vi "rampa_lab2.vi"() -> ()   [LabVIEW 2025]
uses:
  <vilib>/Utility/file.llb/Write Delimited Spreadsheet (DBL).vi
panel:
  out "Bajo":dbl
  out "Alto":dbl
  in  "DC":dbl
  out "Waveform Chart":dynamicdata(graph)
  out "Thermometer":dbl(slide) scale=0.0..100.0
  in  "stop":bool
  # "Duty Cycle [%]"
  # "ALTO:"
  # "BAJO:"
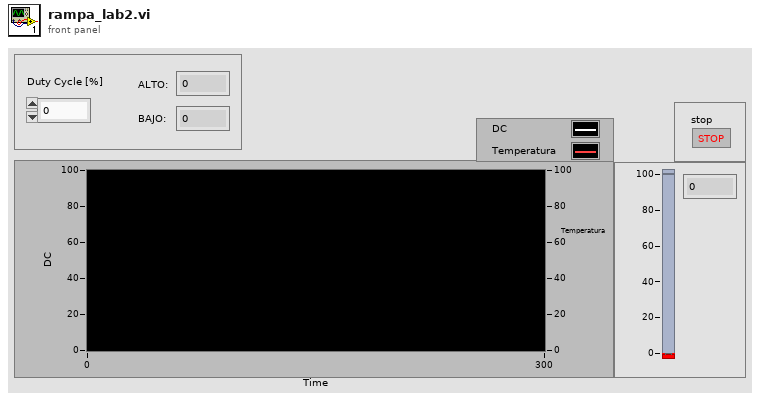
[diagram p1: front panel]
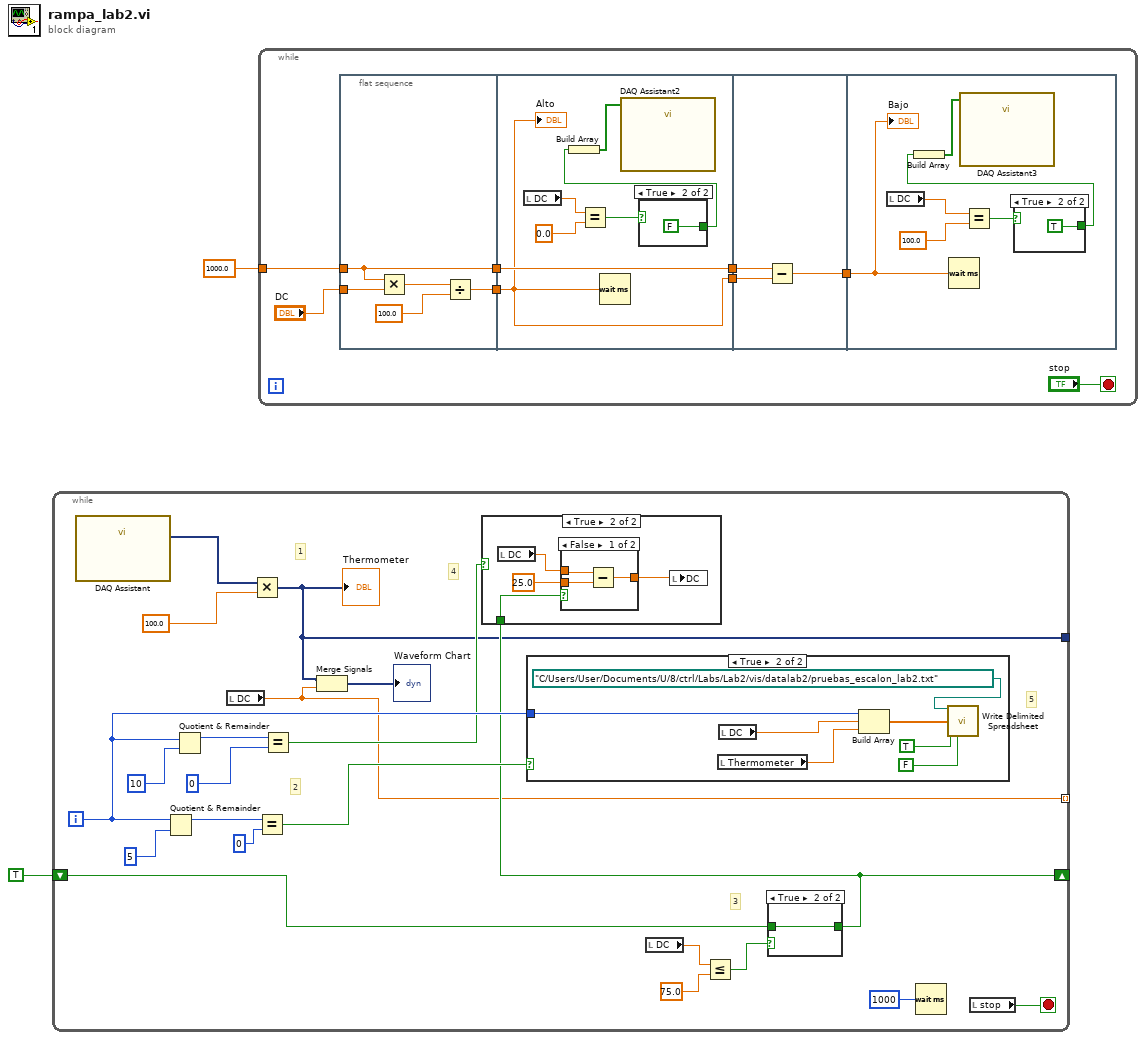
[diagram p0: block diagram]
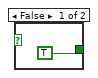
[diagram p2: hidden frame]
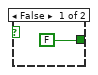
[diagram p3: hidden frame]
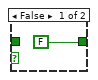
[diagram p4: hidden frame]
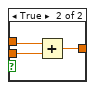
[diagram p6: hidden frame]
diagram:
  n1 = while {
    shift-right: [w7] -> _
    shift-left: TRUE -> [w8]
    tunnel: [w4] -> _
    tunnel: [w3] -> _ mode=indexing
    i -> [w13]
    stop <- w21 stop-if-true
    # "5"
    # "4"
    # "3"
    # "2"
    # "1"
    n2 = call "DAQ Assistant"() -> ("data"=w23:dynamicdata)  [unwired: 17 in, 2 out]
    n3 = Quotient & Remainder(x=w13, y=5) -> (x-y*floor(x/y)=w18:i32)  [unwired: 1 out]
    n4 = Quotient & Remainder(x=w13, y=10) -> (x-y*floor(x/y)=w15:i32)  [unwired: 1 out]
    n5 = local read "DC"() -> (w3:dbl)
    n6 = Multiply(x=w23, y=100.0) -> (x*y=w4:dynamicdata)
    "Thermometer" <- w4
    n7 = Equal?(x=w18, y=0) -> (x = y?=w12:bool)
    n8 = Equal?(x=w15, y=0) -> (x = y?=w6:bool)
    n9 = Merge Signals(w4, w3) -> (→"Waveform Chart":dynamicdata)
    n10 = case shown="True" w12 {
      tunnel: w13 -> [_ w37]
      frame False {
      }
      frame True {
        n11 = local read "Thermometer"() -> (w38:dbl)
        n12 = local read "DC"() -> (w39:dbl)
        n13 = Build Array(w37, w39, w38) -> (w36:dbl[])
        n14 = call-poly <vilib>:"Write Delimited Spreadsheet.vi"("file path (dialog if empty)"=path "C:/Users/User/Documents/U/8/ctrl/Labs/Lab2/vis/datalab2/pruebas_escalon_lab2.txt", "1D data"=w36, "append to file? (new file:F)"=TRUE, "transpose? (no:F)"=FALSE) -> ()  [unwired: 10 in, 2 out]
      }
    }
    n15 = local read "DC"() -> (w10:dbl)
    n16 = Less Or Equal?(x=w10, y=75.0) -> (x <= y?=w9:bool)
    n17 = case shown="True" w9 {
      tunnel: w8 -> [_ w25]
      tunnel: [FALSE w25] -> w7
      frame False {
      }
      frame True {
      }
    }
    n18 = case shown="True" w6 {
      tunnel: w7 -> [_ w29]
      frame False {
      }
      frame True {
        n19 = local read "DC"() -> (w27:dbl)
        n20 = case shown="False" w29 {
          tunnel: 25.0 ("y") -> [w32 w35]
          tunnel: w27 -> [w31 w34]
          tunnel: [w30 w33] -> w26
          frame False {
            n21 = Subtract(x=w31, y=w32) -> (x-y=w30:dbl)
          }
          frame True {
            n22 = Add(x=w34, y=w35) -> (x+y=w33:dbl)
          }
        }
        n23 = local write "DC"(w26) -> ()
      }
    }
    n24 = Wait (ms)(milliseconds to wait=u32 1000) -> ()  [unwired: 1 out]
    n25 = local read "stop"() -> (w21:bool)
  }
  n26 = while {
    tunnel: 1000.0 -> [w49]
    stop <- "stop" stop-if-true
    n27 = flat-sequence {
      tunnel: "DC" -> [w55]
      tunnel: w49 -> [w51]
      tunnel: [w52] -> w48
      tunnel: [w51] -> w47
      tunnel: w48 -> [w60]
      tunnel: w47 -> [w61]
      tunnel: [w61] -> w46
      tunnel: [w60] -> w45
      tunnel: w46 -> [w67]
      tunnel: w45 -> [w66]
      tunnel: [w65] -> w44
      tunnel: w44 -> [w72]
      frame #0 {
        n28 = Multiply(x=w51, y=w55) -> (x*y=w54:dbl)
        n29 = Divide(x=w54, y=100.0) -> (x/y=w52:dbl)
      }
      frame #1 {
        n30 = local read "DC"() -> (w59:dbl)
        n31 = Equal?(x=w59, y=0.0) -> (x = y?=w57:bool)
        n32 = Wait (ms)(milliseconds to wait=w60) -> ()  [unwired: 1 out]
        n33 = case shown="True" w57 {
          tunnel: [TRUE FALSE] -> w56
          frame False {
          }
          frame True {
          }
        }
        n34 = Build Array(w56) -> (w62:bool[])
        n35 = call "DAQ Assistant2"("data"=w62) -> ()  [unwired: 17 in, 2 out]
        "Alto" <- w60
      }
      frame #2 {
        n36 = Subtract(x=w67, y=w66) -> (x-y=w65:dbl)
      }
      frame #3 {
        n37 = local read "DC"() -> (w71:dbl)
        n38 = Wait (ms)(milliseconds to wait=w72) -> ()  [unwired: 1 out]
        n39 = Equal?(x=w71, y=100.0) -> (x = y?=w69:bool)
        n40 = case shown="True" w69 {
          tunnel: [FALSE TRUE] -> w68
          frame False {
          }
          frame True {
          }
        }
        n41 = Build Array(w68) -> (w73:bool[])
        n42 = call "DAQ Assistant3"("data"=w73) -> ()  [unwired: 17 in, 2 out]
        "Bajo" <- w72
      }
    }
  }
